vi "LS218_READ_ETAT_VOIE.vi"(0 "Refnum VISA en entrée":refnum<visa-resource-name>, 1 "numéro voie":i32, 2 "entrée d'erreur (pas d'erreur)":errorcluster) -> (3 "Nom de ressource VISA en sortie":refnum<visa-resource-name>, 4 "Input_ON":bool, 5 "Input_curve":i32, 6 "sortie d'erreur":errorcluster)   [LabVIEW 2016]
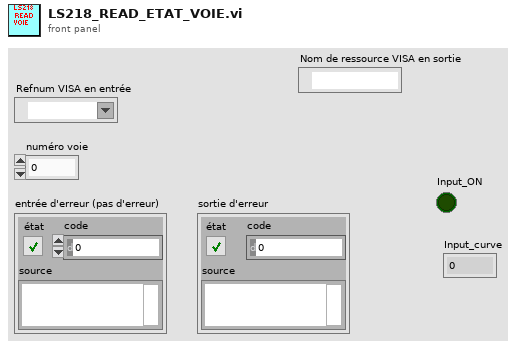
[diagram p1: front panel]
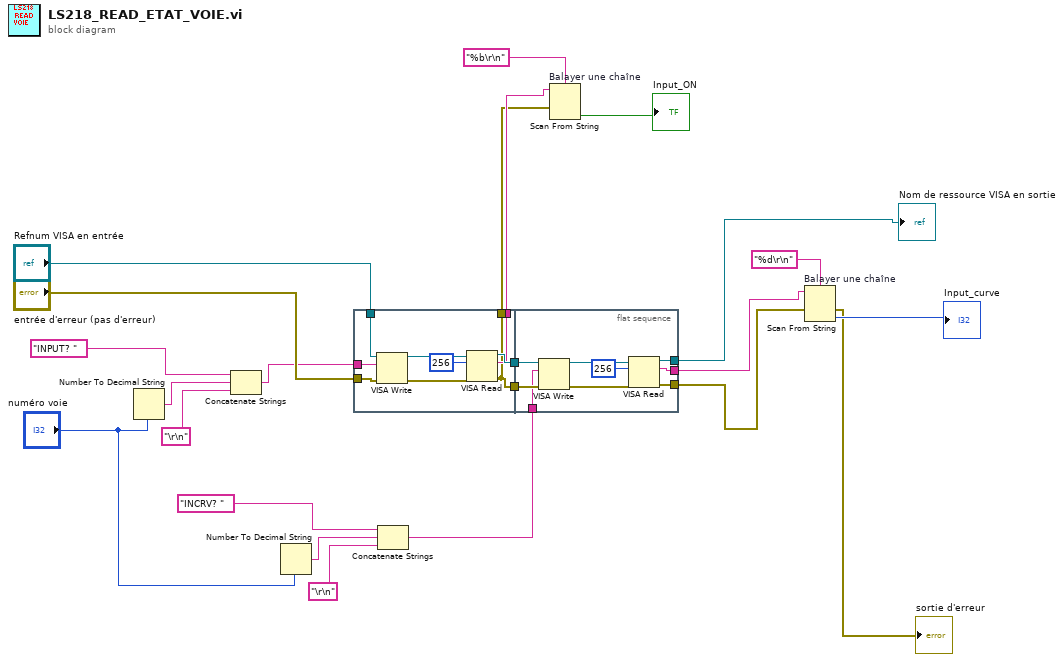
[diagram p0: block diagram]
diagram:
  n1 = Number To Decimal String(number="numéro voie") -> (decimal integer string=w23:string)  [unwired: 1 in]
  n2 = Concatenate Strings("INPUT? " ("chaîne"), w23, "\r\n" ("chaîne")) -> (w3:string)
  n3 = Number To Decimal String(number="numéro voie") -> (decimal integer string=w16:string)  [unwired: 1 in]
  n4 = flat-sequence {
    tunnel: "Refnum VISA en entrée" -> [w29]
    tunnel: "entrée d'erreur (pas d'erreur)" -> [w28]
    tunnel: [w25] -> w7
    tunnel: [w27] -> w6
    tunnel: [w26] -> w5
    tunnel: [w25] -> w4
    tunnel: w3 -> [w24]
    tunnel: [w38] -> w10
    tunnel: [w37] -> w8
    tunnel: [w36] -> w9
    tunnel: w7 -> [w35]
    tunnel: w6 -> [w34]
    tunnel: w2 -> [w33]
    frame #0 {
      n5 = VISA Write(VISA resource name=w29, write buffer=w24, error in (no error)=w28) -> (VISA resource name out=w32:refnum<visa-resource-name>, error out=w31:errorcluster)  [unwired: 1 out]
      n6 = VISA Read(VISA resource name=w32, byte count=u32 256 ("nombre d'octets"), error in (no error)=w31) -> (VISA resource name out=w27:refnum<visa-resource-name>, read buffer=w26:string, error out=w25:errorcluster)  [unwired: 1 out]
    }
    frame #1 {
      n7 = VISA Write(VISA resource name=w34, write buffer=w33, error in (no error)=w35) -> (VISA resource name out=w39:refnum<visa-resource-name>, error out=w40:errorcluster)  [unwired: 1 out]
      n8 = VISA Read(VISA resource name=w39, byte count=u32 256 ("nombre d'octets"), error in (no error)=w40) -> (VISA resource name out=w38:refnum<visa-resource-name>, read buffer=w36:string, error out=w37:errorcluster)  [unwired: 1 out]
    }
  }
  n9 = Concatenate Strings("INCRV? " ("chaîne"), w16, "\r\n" ("chaîne")) -> (w2:string)
  n10 = Scan From String "Balayer une chaîne"(format string="%b\r\n" ("chaîne de format"), input string=w5, error in=w4) -> (output 1=→"Input_ON":bool)  [unwired: 2 in, 3 out]
  n11 = Scan From String "Balayer une chaîne"(format string="%d\r\n" ("chaîne de format"), input string=w9, error in=w8) -> (error out=→"sortie d'erreur":errorcluster, output 1=→"Input_curve":i32)  [unwired: 2 in, 2 out]
  "Nom de ressource VISA en sortie" <- w10
